vi "Template Caller.vi"   [LabVIEW 2019]
uses:
  <extravilib>/ChannelInstances/Event Messenger-c(str,var).lvlib
  <extravilib>/ChannelInstances/Event Messenger-c(str,var)/ChannelOp.ctl
types:
  T1 = typedef "Event Messenger-c(str,var).lvlib/ChannelOp.ctl" = enum16{"init", "write", "register", "replicate", "probe"}
  T2 = typedef "Event Messenger-c(str,var).lvlib/))Channel.ctl" = refnum<queue>
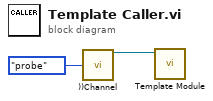
[diagram p0: block diagram]
diagram:
  n1 = call <extravilib>:"))Channel.vi"("channelOp"=ChannelOp."probe") -> ("channel out"=w2:T2)  [unwired: 10 in, 4 out]
  n2 = call "Template Module.vi"("Message Input"=w2) -> ()  [unwired: 10 in, 1 out]
